vi "Actor Core.vi"(8 "error in":errorcluster, 11 "Nested in":refnum<class "User Interface.lvclass">) -> (0 "error out":errorcluster, 3 "Actor out":refnum<class "Actor.lvclass">)   [LabVIEW 2020, in "User Interface.lvlib" / "User Interface.lvclass"]
doc: "(<B>Filename</B>: Actor Framework.lvlib:Actor.lvclass:Actor Core.vi)\n\nReceives messages to the actor, reacts to them, and initiates any error handling that may shut the actor down.\n\nDescendant classes may override this VI to append parallel tasks for the actor to complete while it handles messages. Overrides use the Call Parent Method node."
uses:
  User Interface.lvclass
  C:/Program Files (x86)/National Instruments/LabVIEW 2020/vi.lib/ActorFramework/Actor/Actor.lvclass
  <vilib>/ActorFramework/Actor/Actor.lvclass
  Monedas/Monedas/Monedas.lvclass
  Productos/Productos/Productos.lvclass
  Mensajes/Mensajes/Mensajes.lvclass
  User Interface.lvclass/User Interface.ctl
  <vilib>/ActorFramework/Actor/Actor.lvclass/Actor.ctl
  <vilib>/ActorFramework/Message Enqueuer/Message Enqueuer.lvclass/Message Enqueuer.ctl
  <vilib>/ActorFramework/Message Enqueuer/Init from Existing Queue.vi
  <vilib>/ActorFramework/Message Enqueuer/Enqueue.vi
  <vilib>/ActorFramework/Stop Msg/Stop Msg.lvclass
  C:/Program Files (x86)/National Instruments/LabVIEW 2020/vi.lib/ActorFramework/Message/Message.lvclass
  <vilib>/ActorFramework/Message Priority Queue/Priority Enqueue.vi
  <vilib>/ActorFramework/Message Enqueuer/Message Enqueuer.lvclass
  C:/Users/Pablo/Machine-Vending-AF/User Interface/User Interface.lvclass
panel:
  in  "Producto Agua":bool
  in  "Producto Galletas":bool
  in  "Producto Refresco":bool
  in  "Producto Papas":bool
  in  "Moneda 10":bool
  in  "Moneda 5":bool
  in  "Moneda 2":bool
  in  "Moneda 1":bool
  out "Mensajes":string
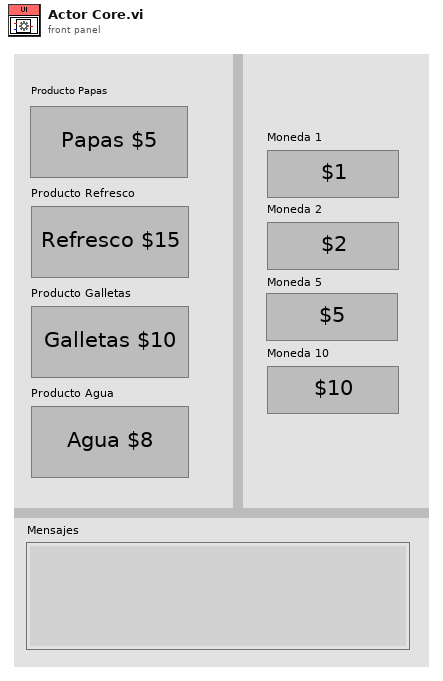
[diagram p1: front panel]
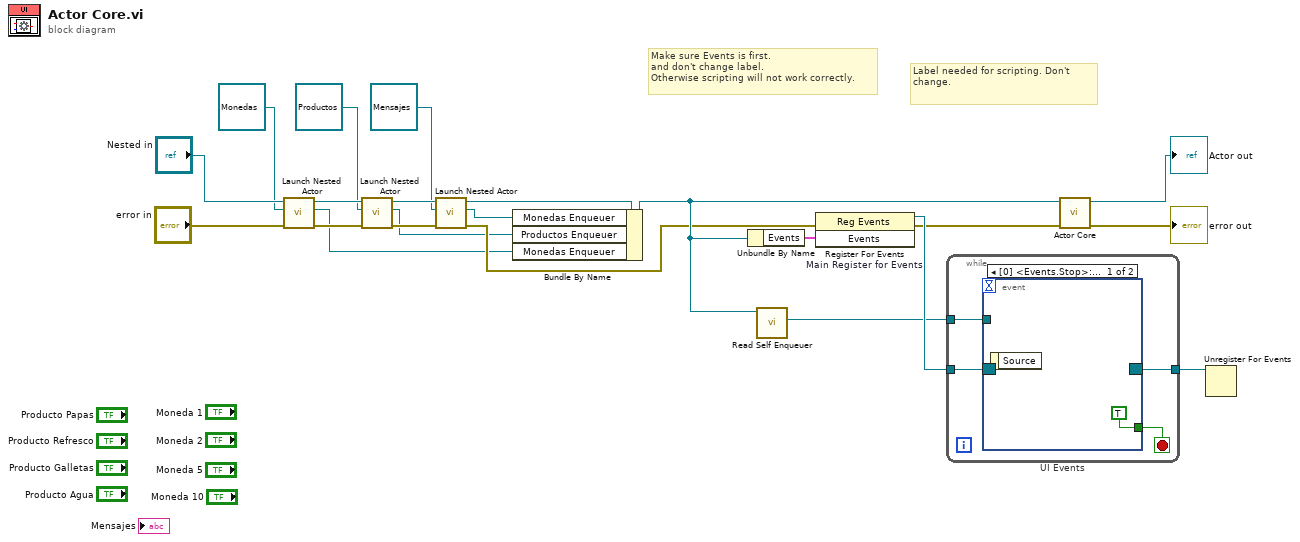
[diagram p0: block diagram]
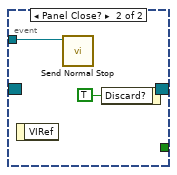
[diagram p2: hidden frame]
diagram:
  # "Label needed for scripting. Don't change."
  # "Make sure Events is first.\nand don't change label.\nOtherwise scripting will not work correctly."
  n1 = call <vilib>:"Launch Nested Actor.vi"("error in (no error)"="error in", "Nested Actor"=refnum<class "Monedas.lvclass"> refnum ("Monedas.lvlib:Monedas.lvclass"), "Caller Actor in"="Nested in") -> ("error out"=w14:errorcluster, "Nested Actor's Enqueuer"=w5:refnum<class "Message Enqueuer.lvclass">, "Caller Actor out"=w9:refnum<class "User Interface.lvclass">)  [unwired: 6 in]
  n2 = call <vilib>:"Launch Nested Actor.vi"("error in (no error)"=w14, "Nested Actor"=refnum<class "Productos.lvclass"> refnum ("Productos.lvlib:Productos.lvclass"), "Caller Actor in"=w9) -> ("error out"=w10:errorcluster, "Nested Actor's Enqueuer"=w3:refnum<class "Message Enqueuer.lvclass">, "Caller Actor out"=w7:refnum<class "User Interface.lvclass">)  [unwired: 6 in]
  n3 = call <vilib>:"Launch Nested Actor.vi"("error in (no error)"=w10, "Nested Actor"=refnum<class "Mensajes.lvclass"> refnum ("Mensajes.lvlib:Mensajes.lvclass"), "Caller Actor in"=w7) -> ("error out"=w8:errorcluster, "Nested Actor's Enqueuer"=w2:refnum<class "Message Enqueuer.lvclass">, "Caller Actor out"=w6:refnum<class "User Interface.lvclass">)  [unwired: 6 in]
  n4 = Bundle By Name(cluster=w6, "Monedas Enqueuer"=w2, "Productos Enqueuer"=w3, "Monedas Enqueuer"=w5) -> (w12:refnum<class "User Interface.lvclass">)
  n5 = Unbundle By Name(w12) -> ("Events"=w19:cluster{"Stop":refnum<user-event>})
  n6 = call <vilib>:"Read Self Enqueuer.vi"("Actor"=w12) -> ("Self Enqueuer"=w17:refnum<class "Message Enqueuer.lvclass">)  [unwired: 10 in]
  n7 = register-events "Main Register for Events"(error in=w8, w19) -> (reference out=w20:refnum<event-registration>, error out=w15:errorcluster)  [unwired: 1 in]
  n8 = while {
    tunnel: w20 -> [w26]
    tunnel: [w24] -> w18
    tunnel: w17 -> [w23]
    stop <- w25 stop-if-true
    n9 = event "UI Events" shown="[0] <Events.Stop>: User Event" {
      selector: w26 -> [_ _]
      dyn-events: [_ _] -> w24
      timeout: _ -> [_ _]
      tunnel: [TRUE _] -> w25
      tunnel: w23 -> [_ w28]
      event User Event {
        n10 = event-data() -> ()  [unwired: 1 in, 1 out]
      }
      event Panel Close? {
        n11 = event-data() -> ()  [unwired: 1 in, 1 out]
        n12 = call <vilib>:"Send Normal Stop.vi"("Message Enqueuer"=w28) -> ()  [unwired: 10 in, 1 out]
        n13 = event-data("Discard?"=TRUE) -> ()  [unwired: 1 in, 1 out]
      }
    }
  }
  n14 = call-parent "Actor Core.vi"("error in"=w15, "Actor in"=w12) -> ("error out"=→"error out":errorcluster, "Actor out"=→"Actor out":refnum<class "Actor.lvclass">)  [unwired: 8 in]
  n15 = Unregister For Events(event registration refnum=w18) -> ()  [unwired: 1 in, 1 out]
